vi "First Identity.vi"(8 "Error In":errorcluster, 10 "Identity In":refnum<class "Agent Identity.lvclass">, 11 "Agent In":refnum<class "Agent.lvclass">) -> (0 "Error Out":errorcluster, 1 "Result":T1 items=["Success", "End of Identities"], 2 "Identity Out":refnum<class "Agent Identity.lvclass">, 3 "Agent Out":refnum<class "Agent.lvclass">)   [LabVIEW 2018, in "Toolkit.lvlib" / "Agent.lvclass"]
doc: "Gets the first identity in the internal libssh2lv shared library linked list of identities obtained from a SSH-agent application. Identities are obtained from a SSH-agent application as a linked list within the libssh2 library. This should be called first, before looping through the linked list with the Next Identity VI."
uses:
  Agent.lvclass
  Type Definitions/Results.ctl
  Agent Identity/Agent Identity.lvclass
  Agent.lvclass/Agent.ctl
  Agent Identity/Agent Identity.lvclass/Agent Identity.ctl
  Session/Session.lvclass/Session.ctl
  SSH/SSH.lvclass/SSH.ctl
  Toolkit.lvlib
  Session/Session.lvclass
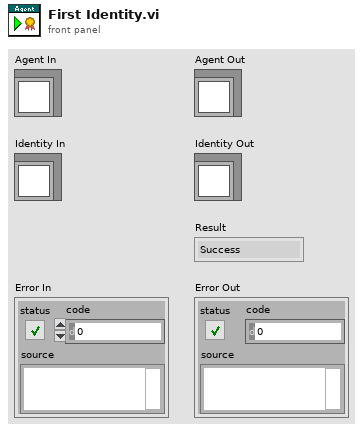
[diagram p1: front panel]
types:
  T1 = typedef "Toolkit.lvlib/Agent.lvclass/Results.ctl" = i32
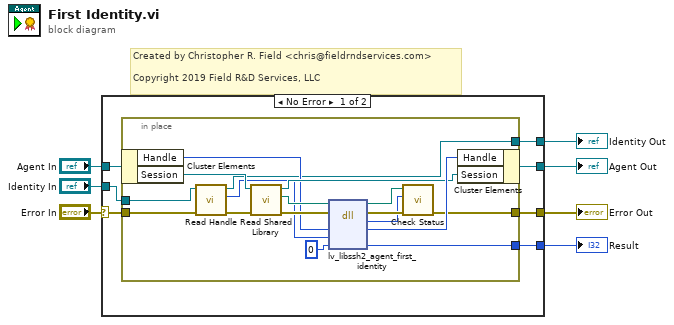
[diagram p0: block diagram]
diagram:
  # "Created by Christopher R. Field <chris@fieldrndservices.com>\n\nCopyright 2019 Field R&D Services, LLC"
  n1 = case shown="No Error" "Error In" {
    selector: "Error In" -> [w14 w34]
    tunnel: [w13 w34] -> w6
    tunnel: "Agent In" -> [w12 w33]
    tunnel: [w11 w33] -> w4
    tunnel: "Identity In" -> [w10 w32]
    tunnel: [w9 w32] -> w2
    tunnel: [w8 _] -> w1
    frame No Error {
      n2 = in-place {
        in-place-border: w14 -> [w19]
        in-place-border: [w28] -> w13
        in-place-border: w10 -> [w20]
        in-place-border: [w17] -> w9
        in-place-border: [w15] -> w8
        n3 = in-place-cluster #1(w12) -> ("Handle"=w22:u64, "Session"=w23:refnum<class "Session.lvclass">)
        n4 = call "Read Handle.vi"("Error In"=w19, "Identity In"=w20) -> ("Error Out"=w18:errorcluster, "Handle"=w16:u64, "Identity Out"=w17:refnum<class "Agent Identity.lvclass">)  [unwired: 7 in]
        n5 = call "Read Shared Library.vi"("Error In"=w18, "Session In"=w23) -> ("Erorr Out"=w26:errorcluster, "libssh2lv Shared Library"=w24:path, "Session Out"=w25:refnum<class "Session.lvclass">)  [unwired: 7 in]
        n6 = dll-call lib="libssh2lv.*" fn="lv_libssh2_agent_first_identity"(path in=w24, error in=w26, "handle"=w22, "identity"=w16, "result"=0) -> (path out=w29:path, error out=w30:errorcluster, "status"=w27:i32, "handle"=w31:u64, "result"=w15:i32)  [unwired: 2 in]
        n7 = call "Check Status.vi"("Error In"=w30, "Status"=w27, "libssh2lv Shared Library In"=w29) -> ("Error Out"=w28:errorcluster)  [unwired: 7 in, 1 out]
        n8 = in-place-cluster #1("Handle"=w31, "Session"=w25) -> (w11:refnum<class "Agent.lvclass">)
      }
    }
    frame Error {
    }
  }
  "Error Out" <- w6
  "Result" <- w1
  "Agent Out" <- w4
  "Identity Out" <- w2
